vi "Display error code.vi"(0 "error in":errorcluster) -> ()   [LabVIEW 2018]
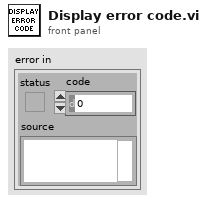
[diagram p1: front panel]
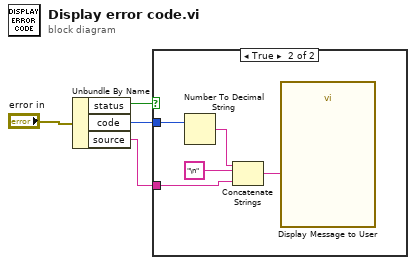
[diagram p0: block diagram]
diagram:
  n1 = Unbundle By Name("error in") -> ("status"=w3:bool, "code"=w2:i32, "source"=w1:string)
  n2 = case shown="True" w3 {
    tunnel: w2 -> [_ w6]
    tunnel: w1 -> [_ w5]
    frame False {
    }
    frame True {
      n3 = Number To Decimal String(number=w6) -> (decimal integer string=w9:string)  [unwired: 1 in]
      n4 = Concatenate Strings(w9, "\n" ("string"), w5) -> (w7:string)
      n5 = call "Display Message to User"("Message"=w7) -> ()  [unwired: 9 in, 2 out]
    }
  }
